vi "Sensors Proccess.vi"(1 "error in":errorcluster) -> ()   [LabVIEW 2013]
uses:
  Sensors Global Values.vi
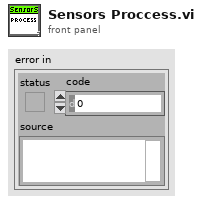
[diagram p1: front panel]
types:
  T1 = cluster{"Camera Sonar":dbl, "Front Right Sonar":dbl, "Front Left Sonar":dbl, "Rear Sonar":dbl}
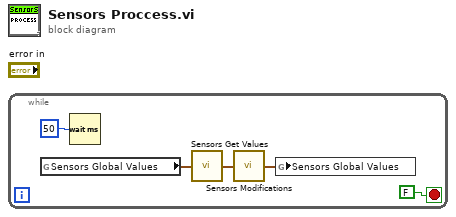
[diagram p0: block diagram]
diagram:
  n1 = while {
    stop <- FALSE stop-if-true
    n2 = global read "Sensors Global Values.vi" "Sensors Global Values"() -> (w3:T1)
    n3 = Wait (ms)(milliseconds to wait=u32 50) -> ()  [unwired: 1 out]
    n4 = call "Sensors Get Values.vi"("Sensors Global Values In"=w3) -> ("Sensors Global Values Out"=w1:T1)
    n5 = call "Sensors Modifications.vi"("Sensors Global Values In"=w1) -> ("Sensors Global Values Out"=w2:T1)
    n6 = global write "Sensors Global Values.vi" "Sensors Global Values"(w2) -> ()
  }
